vi "Start Testing.vi"(8 "error in (no error)":errorcluster, 10 "Test Settings":T1 {"Load Cell Sensitivity" format="%.6f"}, 11 "Context in":refnum<class "Context.lvclass">) -> (0 "error out":errorcluster, 3 "Context out":refnum<class "Context.lvclass">)   [LabVIEW 2016, in "Context.lvclass"]
uses:
  Context.lvclass
  Model/Model/Model.lvclass
  States/State/State.lvclass
  Typedefs/TestSettings.ctl
  Typedefs/HPMT_Typedefs.lvlib
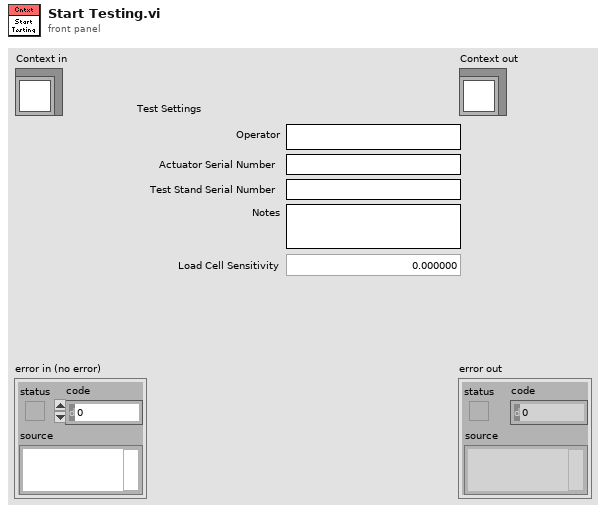
[diagram p1: front panel]
types:
  T1 = typedef "HPMT_Typedefs.lvlib/TestSettings.ctl" = cluster{"Operator":string, "Actuator Serial Number":string, "Test Stand Serial Number":string, "Notes":string, "Load Cell Sensitivity":dbl}
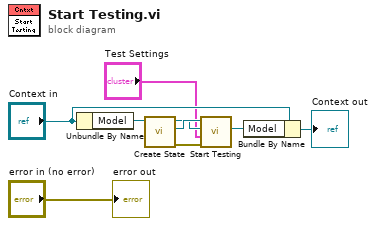
[diagram p0: block diagram]
diagram:
  n1 = Unbundle By Name("Context in") -> ("Model"=w8:refnum<class "Model.lvclass">)
  n2 = call "Create State.vi"("Model in"=w8) -> ("error out"=w2:errorcluster, "State"=w4:refnum<class "State.lvclass">, "Model out"=w3:refnum<class "Model.lvclass">)  [unwired: 8 in]
  n3 = call-dynamic "Start Testing.vi"("error in (no error)"=w2, "Scan Settings"="Test Settings", "Model in"=w3, "State in"=w4) -> ("Model out"=w5:refnum<class "Model.lvclass">)  [unwired: 5 in, 2 out]
  n4 = Bundle By Name(cluster="Context in", "Model"=w5) -> (→"Context out":refnum<class "Context.lvclass">)
  "error out" <- "error in (no error)"
